vi "Abort Scheduled Enqueue.vi"(8 "error in (no error)":errorcluster, 11 "Scheduled Message in":refnum<class "Scheduled Enqueue.lvclass">) -> (0 "error out":errorcluster)   [LabVIEW 2020, in "Scheduled Enqueue.lvclass"]
uses:
  Scheduled Enqueue.lvclass
  Scheduled Enqueue.lvclass/Scheduled Enqueue.ctl
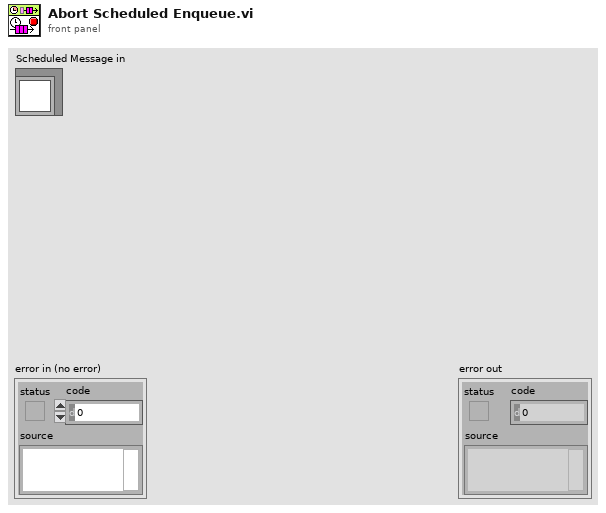
[diagram p1: front panel]
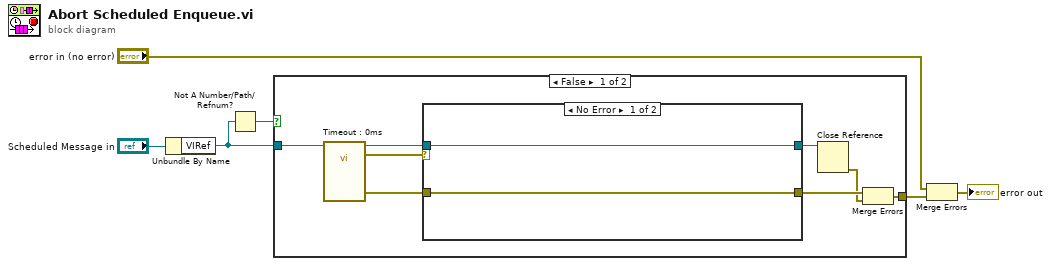
[diagram p0: block diagram]
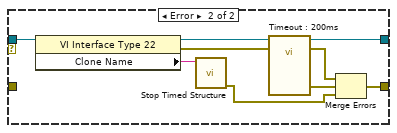
[diagram p2: hidden frame]
diagram:
  n1 = Unbundle By Name("Scheduled Message in") -> ("VIRef"=w4:refnum<vi>)
  n2 = Not A Number/Path/Refnum?(number/path/refnum=w4) -> (NaN/Path/Refnum?=w3:bool)
  n3 = case shown="False" w3 {
    tunnel: [w14 _] -> w6
    tunnel: w4 -> [w7 _]
    frame False {
      n4 = call-by-ref "Timeout : 0ms"(reference=w7) -> (reference out=w13:refnum<vi>, error out=w12:errorcluster, 0:"error out"=w11:errorcluster)  [unwired: 12 in]
      n5 = case shown="No Error" w12 {
        tunnel: w13 -> [w16 w25]
        tunnel: w11 -> [w15 _]
        tunnel: [w16 w22] -> w9
        tunnel: [w15 w19] -> w10
        frame No Error {
        }
        frame Error {
          n6 = property class="VI Interface Type 22"(reference=w25) -> (reference out=w23:refnum<vi>, error out=w21:errorcluster, "Clone Name"=w24:string)  [unwired: 1 in]
          n7 = call <vilib>:"Stop Timed Structure.vi"("name"=w24) -> ("error out"=w20:errorcluster)  [unwired: 10 in]
          n8 = call-by-ref "Timeout : 200ms"(reference=w23, error in=w21) -> (reference out=w22:refnum<vi>, error out=w17:errorcluster, 0:"error out"=w18:errorcluster)  [unwired: 11 in]
          n9 = Merge Errors(w17, w18, w20) -> (w19:errorcluster)
        }
      }
      n10 = Close Reference(reference=w9) -> (error out=w8:errorcluster)  [unwired: 1 in]
      n11 = Merge Errors(w10, w8) -> (w14:errorcluster)
    }
    frame True {
    }
  }
  n12 = Merge Errors("error in (no error)", w6) -> (→"error out":errorcluster)
